vi "String To Sensor Bits.vi"(8 "error in (no error)":errorcluster caption="错误输入（无错误）", 9 "autoDetectAsicType":i32, 10 "pszSourceBuffer":string, 11 "sensorHandle":i32) -> (0 "error out":errorcluster caption="错误输出", 2 "pszSourceBuffer out":string, 3 "function return":i32)   [LabVIEW 2018]
doc: "extern int __stdcall APSxStringToSensorBits (int sensorHandle, IN char pszSourceBuffer[], IN int autoDetectAsicType);"
uses:
  APSx.dll/APSx.dll
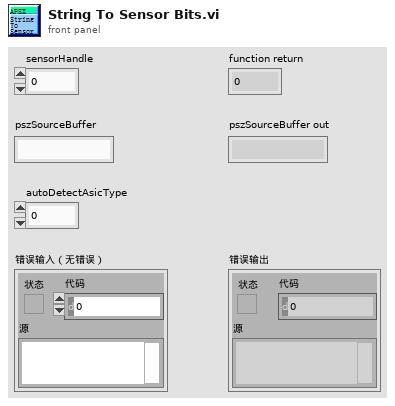
[diagram p1: front panel]
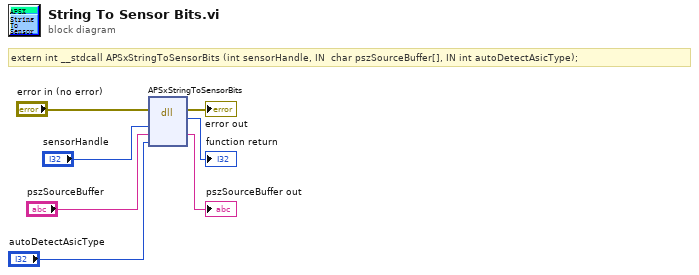
[diagram p0: block diagram]
diagram:
  # "extern int __stdcall APSxStringToSensorBits (int sensorHandle, IN  char pszSourceBuffer[], IN int autoDetectAsicType);"
  n1 = dll-call lib="PTH2[abs D项目Feng恒隆项目Labview传感器对中台SourcesAPSx.dllAPSx.*" fn="APSxStringToSensorBits"(error in="error in (no error)", "sensorHandle"="sensorHandle", "pszSourceBuffer"="pszSourceBuffer", "autoDetectAsicType"="autoDetectAsicType") -> (error out=→"error out":errorcluster, →"function return":i32, "pszSourceBuffer"=→"pszSourceBuffer out":string)  [unwired: 4 in, 1 out]
